vi "Game mode.vi"() -> ()   [LabVIEW 2019]
uses:
  Global 8.vi
panel:
  in  "start game":bool
  out "String 2":string
  out "String":string
  in  "Player 1":string
  in  "Player 2":string
  in  "Player 3":string
  in  "Player 4":string
  in  "4 Players":bool
  in  "3 Players":bool
  in  "2 Players":bool
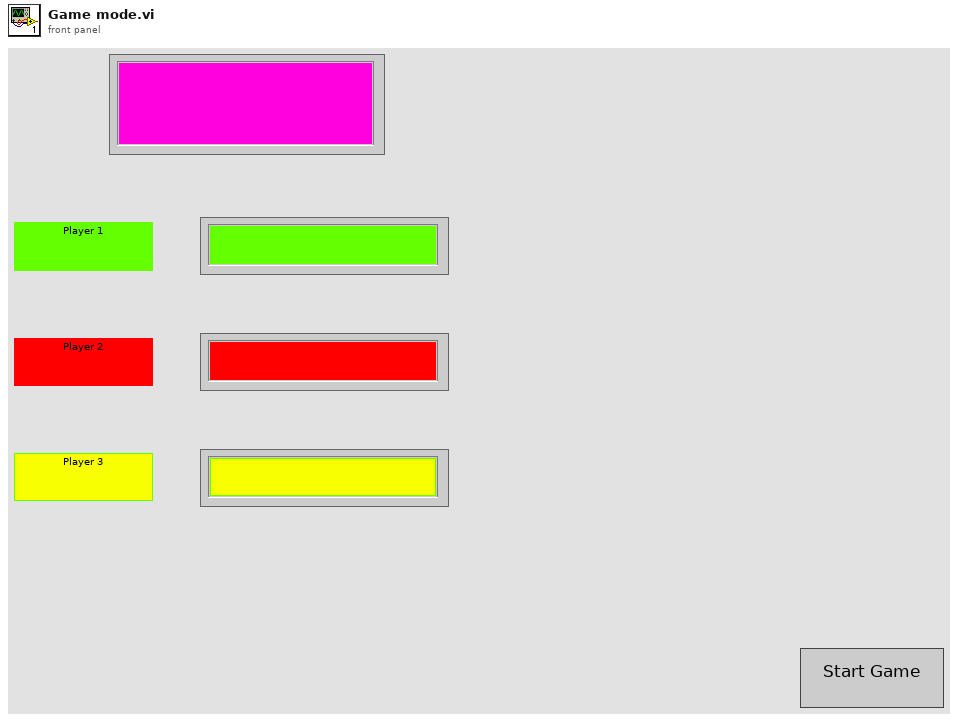
[diagram p1: front panel]
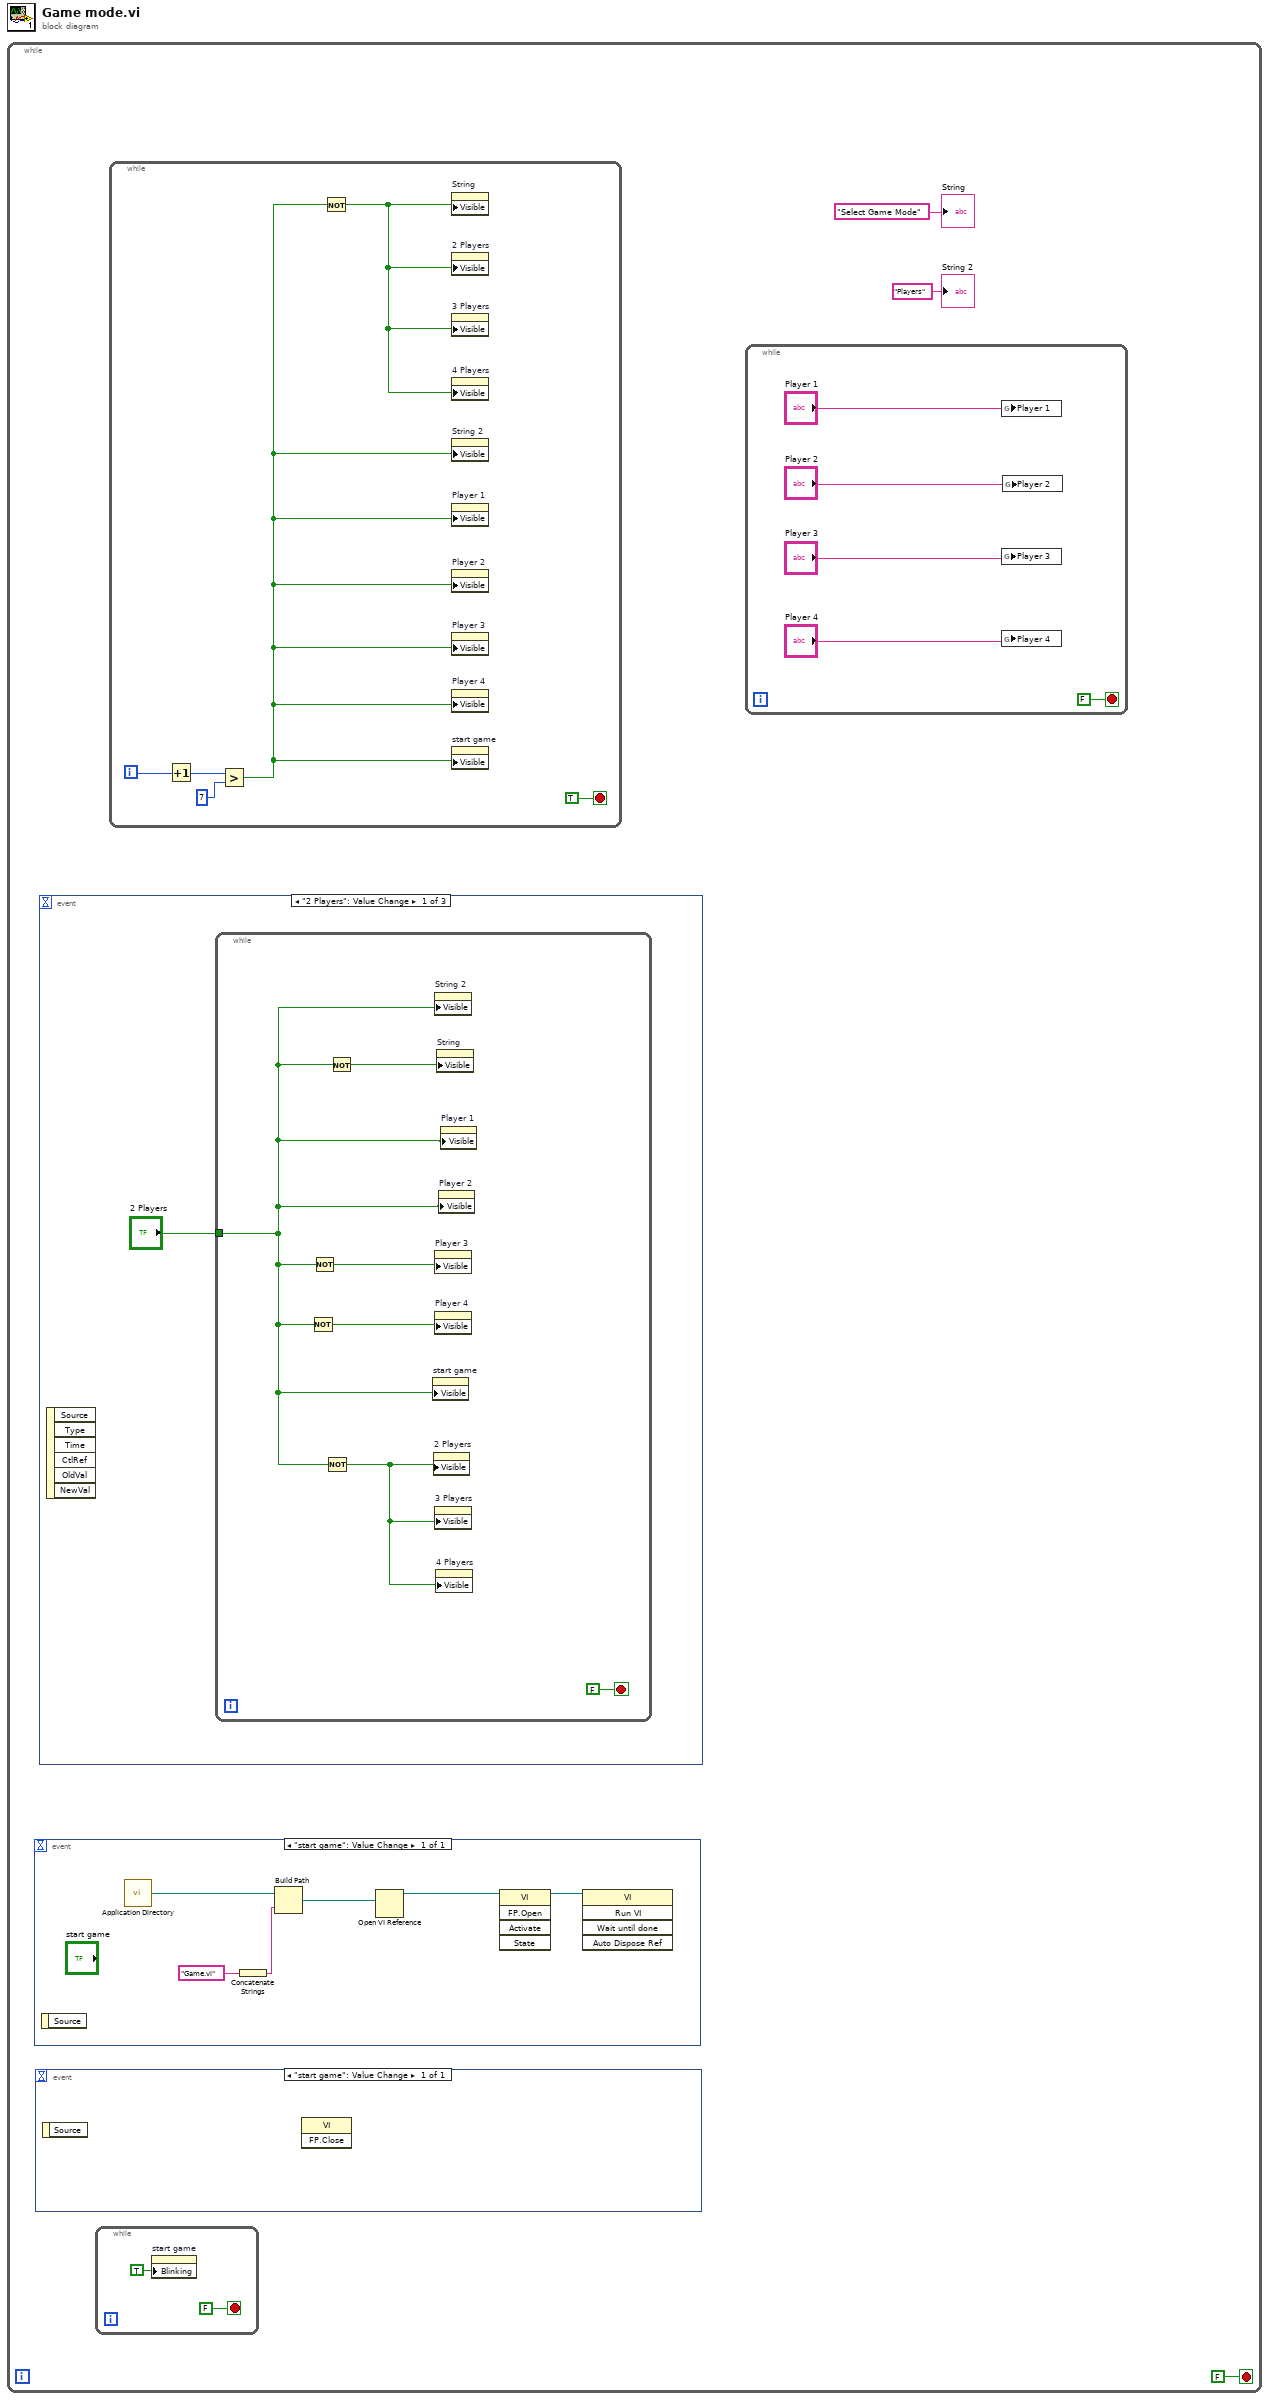
[diagram p0: block diagram]
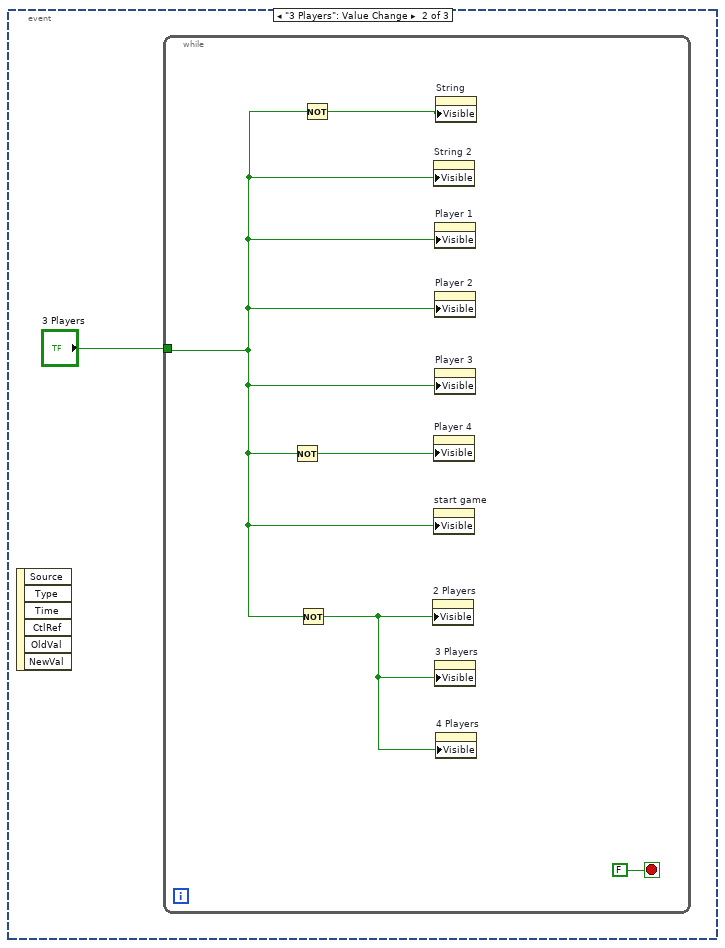
[diagram p2: hidden frame]
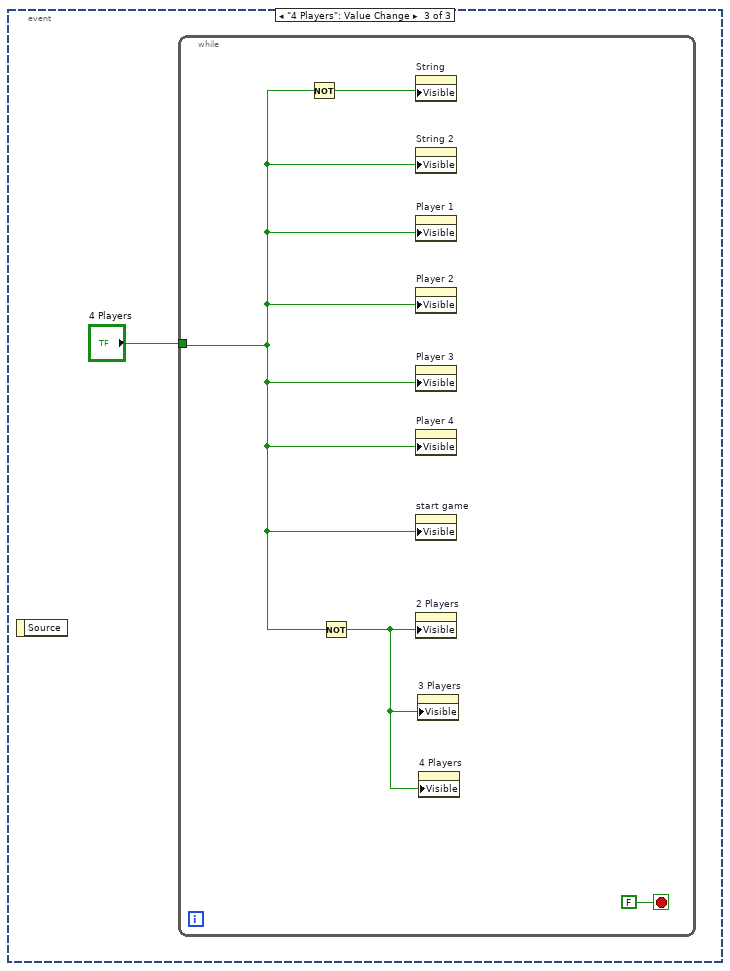
[diagram p3: hidden frame]
diagram:
  n1 = while {
    stop <- FALSE stop-if-true
    n2 = event shown="[0] \"start game\": Value Change" {
      selector: _ -> [_]
      dyn-events: _ -> [_]
      timeout: _ -> [_]
      event "start game": Value Change {
        n3 = event-data() -> ()  [unwired: 1 in, 1 out]
        n4 = call <vilib>:"Application Directory.vi"() -> ("Application Directory"=w38:path)
        n5 = Concatenate Strings("Game.vi" ("string")) -> (w37:string)
        n6 = Build Path(base path=w38, name or relative path=w37) -> (appended path=w35:path)
        n7 = Open VI Reference(vi path=w35) -> (vi reference=w34:refnum<vi>)  [unwired: 5 in, 1 out]
        n8 = invoke class="VI" method="FP.Open"(reference=w34) -> (reference out=w33:refnum<vi>)  [unwired: 4 in, 4 out]
        n9 = invoke class="VI" method="Run VI"(reference=w33) -> ()  [unwired: 4 in, 5 out]
      }
    }
    n10 = event shown="[0] \"start game\": Value Change" {
      selector: _ -> [_]
      dyn-events: _ -> [_]
      timeout: _ -> [_]
      event "start game": Value Change {
        n11 = event-data() -> ()  [unwired: 1 in, 1 out]
        n12 = invoke class="VI" method="FP.Close"() -> ()  [unwired: 3 in, 3 out]
      }
    }
    n13 = event shown="[0] \"2 Players\": Value Change" {
      selector: _ -> [_ _ _]
      dyn-events: _ -> [_ _ _]
      timeout: _ -> [_ _ _]
      event "2 Players": Value Change {
        n14 = event-data() -> ()  [unwired: 1 in, 6 out]
        n15 = while {
          tunnel: "2 Players" -> [w16]
          stop <- FALSE stop-if-true
          n16 = Not(x=w16) -> (.not. x?=w19:bool)
          n17 = Not(x=w16) -> (.not. x?=w20:bool)
          n18 = Not(x=w16) -> (.not. x?=w17:bool)
          n19 = Not(x=w16) -> (.not. x?=w18:bool)
          n20 = property on="start game" class="Bool"("Visible"=w16) -> ()  [unwired: 2 in, 2 out]
          n21 = property on="2 Players" class="Bool"("Visible"=w17) -> ()  [unwired: 2 in, 2 out]
          n22 = property on="String 2" class="Str"("Visible"=w16) -> ()  [unwired: 2 in, 2 out]
          n23 = property on="Player 3" class="Str"("Visible"=w20) -> ()  [unwired: 2 in, 2 out]
          n24 = property on="Player 4" class="Str"("Visible"=w19) -> ()  [unwired: 2 in, 2 out]
          n25 = property on="3 Players" class="Bool"("Visible"=w17) -> ()  [unwired: 2 in, 2 out]
          n26 = property on="4 Players" class="Bool"("Visible"=w17) -> ()  [unwired: 2 in, 2 out]
          n27 = property on="String" class="Str"("Visible"=w18) -> ()  [unwired: 2 in, 2 out]
          n28 = property on="Player 2" class="Str"("Visible"=w16) -> ()  [unwired: 2 in, 2 out]
          n29 = property on="Player 1" class="Str"("Visible"=w16) -> ()  [unwired: 2 in, 2 out]
        }
      }
      event "3 Players": Value Change {
        n30 = event-data() -> ()  [unwired: 1 in, 6 out]
        n31 = while {
          tunnel: "3 Players" -> [w23]
          stop <- FALSE stop-if-true
          n32 = Not(x=w23) -> (.not. x?=w26:bool)
          n33 = Not(x=w23) -> (.not. x?=w24:bool)
          n34 = Not(x=w23) -> (.not. x?=w25:bool)
          n35 = property on="2 Players" class="Bool"("Visible"=w24) -> ()  [unwired: 2 in, 2 out]
          n36 = property on="String 2" class="Str"("Visible"=w23) -> ()  [unwired: 2 in, 2 out]
          n37 = property on="Player 4" class="Str"("Visible"=w26) -> ()  [unwired: 2 in, 2 out]
          n38 = property on="start game" class="Bool"("Visible"=w23) -> ()  [unwired: 2 in, 2 out]
          n39 = property on="Player 1" class="Str"("Visible"=w23) -> ()  [unwired: 2 in, 2 out]
          n40 = property on="Player 2" class="Str"("Visible"=w23) -> ()  [unwired: 2 in, 2 out]
          n41 = property on="Player 3" class="Str"("Visible"=w23) -> ()  [unwired: 2 in, 2 out]
          n42 = property on="3 Players" class="Bool"("Visible"=w24) -> ()  [unwired: 2 in, 2 out]
          n43 = property on="String" class="Str"("Visible"=w25) -> ()  [unwired: 2 in, 2 out]
          n44 = property on="4 Players" class="Bool"("Visible"=w24) -> ()  [unwired: 2 in, 2 out]
        }
      }
      event "4 Players": Value Change {
        n45 = event-data() -> ()  [unwired: 1 in, 1 out]
        n46 = while {
          tunnel: "4 Players" -> [w30]
          stop <- FALSE stop-if-true
          n47 = Not(x=w30) -> (.not. x?=w31:bool)
          n48 = Not(x=w30) -> (.not. x?=w29:bool)
          n49 = property on="String" class="Str"("Visible"=w31) -> ()  [unwired: 2 in, 2 out]
          n50 = property on="String 2" class="Str"("Visible"=w30) -> ()  [unwired: 2 in, 2 out]
          n51 = property on="Player 1" class="Str"("Visible"=w30) -> ()  [unwired: 2 in, 2 out]
          n52 = property on="Player 2" class="Str"("Visible"=w30) -> ()  [unwired: 2 in, 2 out]
          n53 = property on="Player 3" class="Str"("Visible"=w30) -> ()  [unwired: 2 in, 2 out]
          n54 = property on="Player 4" class="Str"("Visible"=w30) -> ()  [unwired: 2 in, 2 out]
          n55 = property on="start game" class="Bool"("Visible"=w30) -> ()  [unwired: 2 in, 2 out]
          n56 = property on="2 Players" class="Bool"("Visible"=w29) -> ()  [unwired: 2 in, 2 out]
          n57 = property on="3 Players" class="Bool"("Visible"=w29) -> ()  [unwired: 2 in, 2 out]
          n58 = property on="4 Players" class="Bool"("Visible"=w29) -> ()  [unwired: 2 in, 2 out]
        }
      }
    }
    n59 = while {
      stop <- FALSE stop-if-true
      n60 = property on="start game" class="Bool"("Blinking"=TRUE) -> ()  [unwired: 2 in, 2 out]
    }
    n61 = while {
      i -> [w11]
      stop <- TRUE stop-if-true
      n62 = Increment(x=w11) -> (x+1=w12:i32)
      n63 = Greater?(x=w12, y=7) -> (0:w9:bool)
      n64 = Not(x=w9) -> (.not. x?=w10:bool)
      n65 = property on="String" class="Str"("Visible"=w10) -> ()  [unwired: 2 in, 2 out]
      n66 = property on="2 Players" class="Bool"("Visible"=w10) -> ()  [unwired: 2 in, 2 out]
      n67 = property on="3 Players" class="Bool"("Visible"=w10) -> ()  [unwired: 2 in, 2 out]
      n68 = property on="4 Players" class="Bool"("Visible"=w10) -> ()  [unwired: 2 in, 2 out]
      n69 = property on="String 2" class="Str"("Visible"=w9) -> ()  [unwired: 2 in, 2 out]
      n70 = property on="Player 1" class="Str"("Visible"=w9) -> ()  [unwired: 2 in, 2 out]
      n71 = property on="Player 2" class="Str"("Visible"=w9) -> ()  [unwired: 2 in, 2 out]
      n72 = property on="Player 3" class="Str"("Visible"=w9) -> ()  [unwired: 2 in, 2 out]
      n73 = property on="Player 4" class="Str"("Visible"=w9) -> ()  [unwired: 2 in, 2 out]
      n74 = property on="start game" class="Bool"("Visible"=w9) -> ()  [unwired: 2 in, 2 out]
    }
    n75 = while {
      stop <- FALSE stop-if-true
      n76 = global write "Global 8.vi" "Player 1"("Player 1") -> ()
      n77 = global write "Global 8.vi" "Player 3"("Player 3") -> ()
      n78 = global write "Global 8.vi" "Player 4"("Player 4") -> ()
      n79 = global write "Global 8.vi" "Player 2"("Player 2") -> ()
    }
    "String" <- "Select Game Mode" ("String")
    "String 2" <- "Players" ("String 2")
  }
